vi "Create Simple Template file.vi"(2 "Wanted Channels":string[](array[string]), 3 "Template File":path) -> ()   [LabVIEW 2022 SP3]
uses:
  Controls/Global_mode.ctl
  File_Template_Clus.ctl
  Data plotting/subVIs/Dispose_Channel.ctl
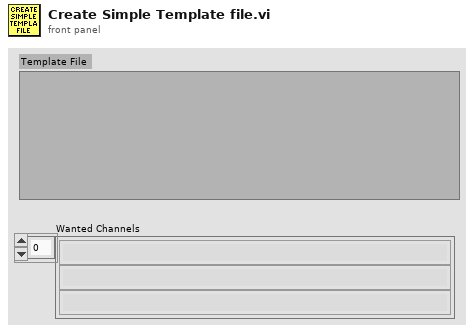
[diagram p1: front panel]
types:
  T1 = typedef "Dispose_Channel.ctl" = enum16{"Always", "If Blank", "Never"}
  T2 = typedef "File_Template_Clus.ctl" = cluster{"Template Channel Name":string, "Description":string, "Tolerance":dbl, "Precision":string, "Folder level":string, "Source":string[], "Replace":string[], "Summarise":bool, "Min Value":string, "Maths":string, "Omit Rows Containing":string[], "Ignore When":string[], "Max Value":string, "Dispose":T1}
  T3 = typedef "Global_mode.ctl" = enum16{"Read Global", "Load Global From File", "Write Global to File"}
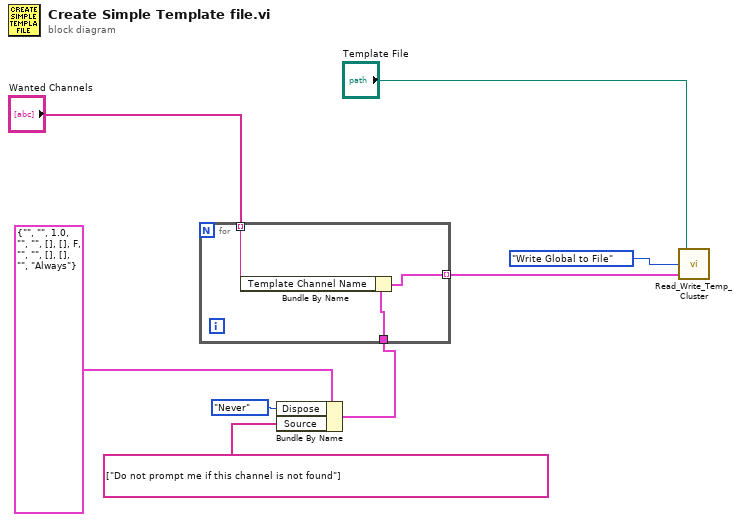
[diagram p0: block diagram]
diagram:
  n1 = Bundle By Name(cluster=T2 {"Template Channel Name"="", "Description"="", "Tolerance"=1.0, "Precision"="", "Folder level"="", "Source"=[], "Replace"=[], "Summarise"=FALSE, "Min Value"="", "Maths"="", "Omit Rows Containing"=[], "Ignore When"=[], "Max Value"="", "Dispose"=enum."Always"} ("Cluster"), "Dispose"=Dispose_Channel."Never", "Source"=string[] ["Do not prompt me if this channel is not found"]) -> (w3:T2)
  n2 = for {
    tunnel: w3 -> [w11]
    tunnel: "Wanted Channels" -> [w10] mode=indexing
    tunnel: [w9] -> w6 mode=indexing
    n3 = Bundle By Name(cluster=w11, "Template Channel Name"=w10) -> (w9:T2)
  }
  n4 = call "Read_Write_Temp_Cluster.vi"("Template Info Array"=w6, "Mode"=Global_mode."Write Global to File", "Template File"="Template File") -> ()  [unwired: 3 out]
